vi "FE ID to D-Simulated ID.vi"(1 "Opt H?":bool, 2 "Opt F?":bool, 3 "Opt. D?":bool, 7 "B-series ID":i32) -> (8 "Config 'D' ID":i32)   [LabVIEW 2011]
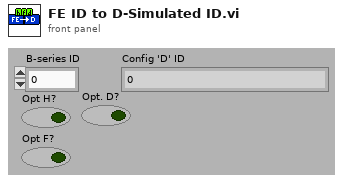
[diagram p1: front panel]
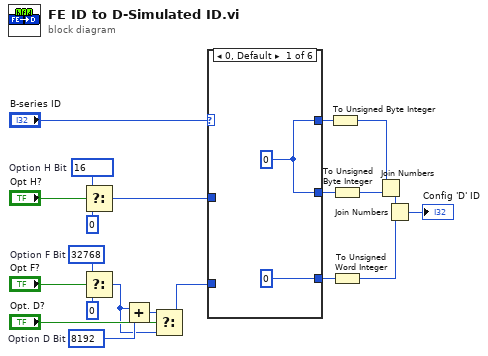
[diagram p0: block diagram]
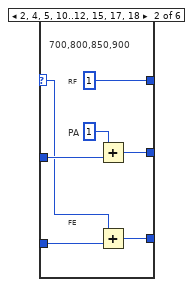
[diagram p2: hidden frame]
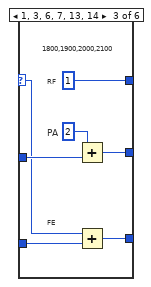
[diagram p3: hidden frame]
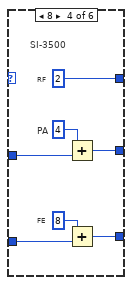
[diagram p4: hidden frame]
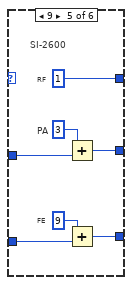
[diagram p5: hidden frame]
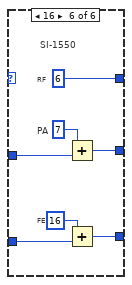
[diagram p6: hidden frame]
diagram:
  w8 = u16 8192  # Option D Bit
  w15 = u16 32768  # Option F Bit
  w20 = u8 16  # Option H Bit
  n1 = Select(t=w20, s="Opt H?", f=u8 0) -> (s? t:f=w17:u8)
  n2 = Select(t=w15, s="Opt F?", f=u16 0) -> (s? t:f=w5:u16)
  n3 = Add(x=w5, y=w8) -> (x+y=w6:u16)
  n4 = Select(t=w6, s="Opt. D?", f=w5) -> (s? t:f=w4:u16)
  n5 = case shown="0, Default" "B-series ID" {
    selector: "B-series ID" -> [_ w24 w31 _ _ _]
    tunnel: w17 -> [_ w29 w36 w40 w47 w54]
    tunnel: w4 -> [_ w30 w37 w39 w46 w53]
    tunnel: [w23 u8 1 ("RF") u8 1 ("RF") u8 2 ("RF") u8 1 ("RF") u8 6 ("RF")] -> w10
    tunnel: [w23 w26 w33 w41 w48 w55] -> w11
    tunnel: [u16 0 ("FE") w25 w32 w38 w45 w52] -> w12
    frame 0, Default {
      w23 = u8 0
    }
    frame 2, 4, 5, 10..12, 15, 17, 18 {
      # "FE"
      # "PA"
      # "RF"
      # "700,800,850,900"
      n6 = Add(x=u8 1 ("RF"), y=w29) -> (x+y=w26:u8)
      n7 = Add(x=w24, y=w30) -> (x+y=w25:i32)
    }
    frame 1, 3, 6, 7, 13, 14 {
      # "FE"
      # "PA"
      # "RF"
      # "1800,1900,2000,2100"
      n8 = Add(x=u8 2 ("RF"), y=w36) -> (x+y=w33:u8)
      n9 = Add(x=w31, y=w37) -> (x+y=w32:i32)
    }
    frame 8 {
      # "FE"
      # "PA"
      # "RF"
      # "SI-3500"
      n10 = Add(x=u8 4 ("RF"), y=w40) -> (x+y=w41:u8)
      n11 = Add(x=u16 8 ("FE"), y=w39) -> (x+y=w38:u16)
    }
    frame 9 {
      # "FE"
      # "PA"
      # "RF"
      # "SI-2600"
      n12 = Add(x=u8 3 ("RF"), y=w47) -> (x+y=w48:u8)
      n13 = Add(x=u16 9 ("FE"), y=w46) -> (x+y=w45:u16)
    }
    frame 16 {
      # "FE"
      # "PA"
      # "RF"
      # "SI-1550"
      n14 = Add(x=u8 7 ("RF"), y=w54) -> (x+y=w55:u8)
      n15 = Add(x=u16 16 ("FE"), y=w53) -> (x+y=w52:u16)
    }
  }
  n16 = To Unsigned Byte Integer(number=w10) -> (unsigned 8bit integer=w3:u8)
  n17 = To Unsigned Byte Integer(number=w11) -> (unsigned 8bit integer=w2:u8)
  n18 = To Unsigned Word Integer(number=w12) -> (unsigned 16bit integer=w1:u16)
  n19 = Join Numbers(hi=w3, lo=w2) -> ((hi.lo)=w13:u16)
  n20 = Join Numbers(hi=w13, lo=w1) -> ((hi.lo)=→"Config 'D' ID":u32)
